vi "Send Register Actor.vi"(8 "error in (no error)":errorcluster, 9 "Details":T1, 10 "Debug Alias":string, 11 "Message Enqueuer":refnum<class "Message Enqueuer.lvclass">) -> (0 "error out":errorcluster, 3 "Message Enqueuer out":refnum<class "Message Enqueuer.lvclass">)   [LabVIEW 2020, in "AF Debug.lvlib" / "Register Actor Msg.lvclass"]
doc: "This VI sends the message to any actor to tell that actor to register its Actor Core clone name with the debugging tools."
uses:
  Register Actor Msg.lvclass
  vi.lib/ActorFramework/Message Enqueuer/Message Enqueuer.lvclass
  C:/dev/actor-framework/dist/vi.lib/ActorFramework/Message/Message.lvclass
  Register Actor Msg.lvclass/Register Actor Msg.ctl
  vi.lib/ActorFramework/Message Enqueuer/Message Enqueuer.lvclass/Message Enqueuer.ctl
  vi.lib/ActorFramework/Message Enqueuer/Message Priority.ctl
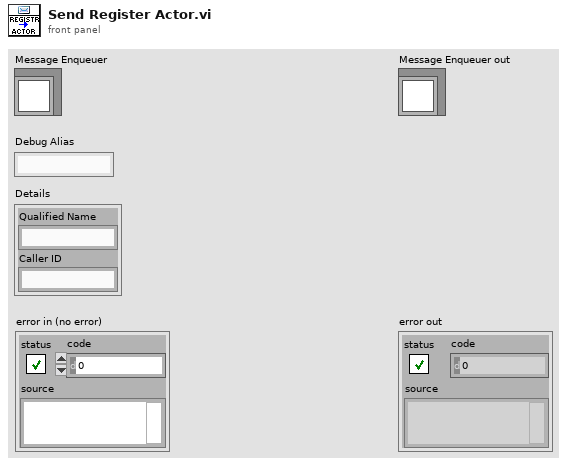
[diagram p1: front panel]
types:
  T1 = cluster{"Qualified Name":string, "Caller ID":string}
  T2 = typedef "Actor Framework.lvlib/Message Enqueuer.lvclass/Message Priority.ctl" = enum16{"Low", "Normal", "High"}
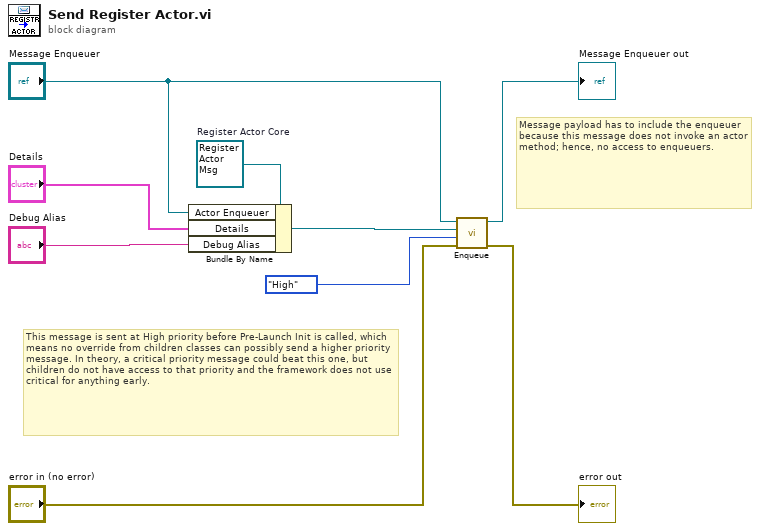
[diagram p0: block diagram]
diagram:
  w5 = refnum<class "Register Actor Msg.lvclass"> refnum  # Register Actor Core
  # "Message payload has to include the enqueuer because this message does not invoke an actor method; hence, no access to enqueuers."
  # "This message is sent at High priority before Pre-Launch Init is called, which means no override from children classes can possibly send a higher priority message. In theory, a critical priority message could beat this one, but children do not have access to that priority and the framework does not use critical for anything early."
  n1 = Bundle By Name(cluster=w5, "Actor Enqueuer"="Message Enqueuer", "Details"="Details", "Debug Alias"="Debug Alias") -> (w4:refnum<class "Register Actor Msg.lvclass">)
  n2 = call "Enqueue.vi"("error in (no error)"="error in (no error)", "Message Priority (Normal)"=Message_Priority."High", "Message"=w4, "Message Enqueuer in"="Message Enqueuer") -> ("error out"=→"error out":errorcluster, "Message Enqueuer out"=→"Message Enqueuer out":refnum<class "Message Enqueuer.lvclass">)  [unwired: 6 in]
